vi "Newmark-CatchCharacters.vi"(0 "Table VRN IN":refnum<visa-resource-name>, 2 "Bool Refnum":refnum<vi>, 11 "Error IN":errorcluster) -> (4 "Table VRN OUT":refnum<visa-resource-name>, 6 "n_chars":u32, 10 "InterruptType":i32(ring) items=["Unknown"=-1, "Error"=0, "Slip/Stall"=1, "Overtravel"=2, "Done"=3, "None"=4], 15 "Error OUT":errorcluster)   [LabVIEW 2011]
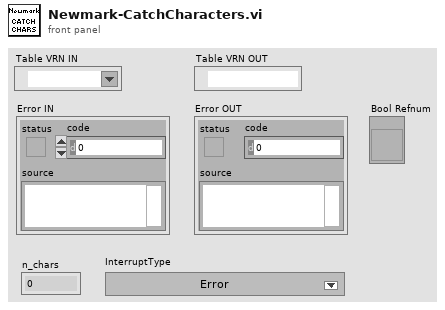
[diagram p1: front panel]
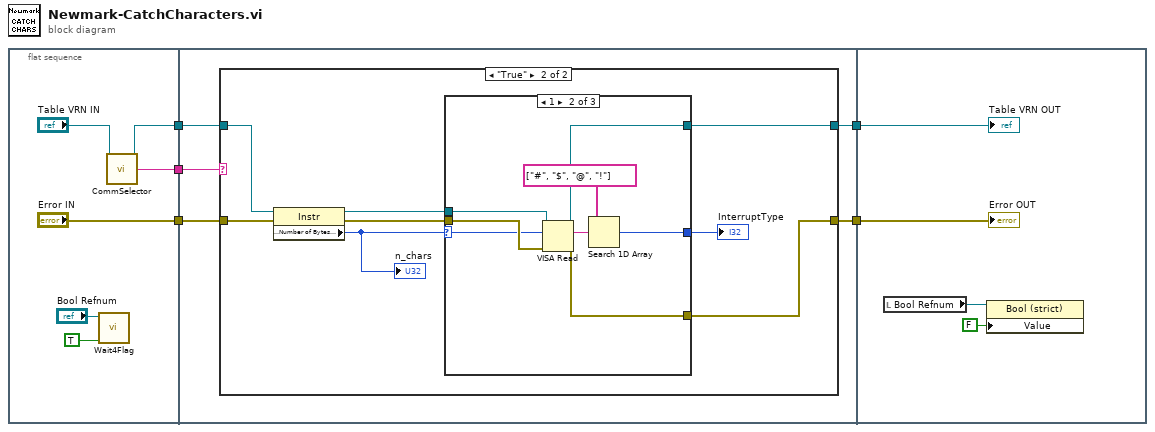
[diagram p0: block diagram]
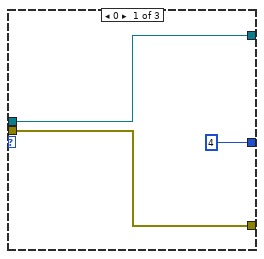
[diagram p3: hidden frame]
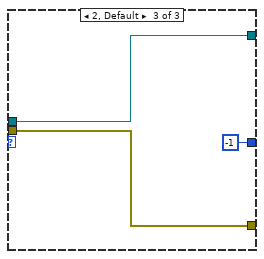
[diagram p4: hidden frame]
diagram:
  n1 = flat-sequence {
    tunnel: ["Error IN"] -> w5
    tunnel: [w7] -> w4
    tunnel: [w6] -> w3
    tunnel: w5 -> [w14]
    tunnel: w4 -> [w16]
    tunnel: w3 -> [w15]
    tunnel: [w13] -> w2
    tunnel: [w12] -> w1
    tunnel: w2 -> [w42]
    tunnel: w1 -> [w41]
    frame #0 {
      n2 = call "Wait4Flag.vi"("Raise Flag ?"=TRUE, "Ctl Refnum IN"="Bool Refnum") -> ()  [unwired: 8 in, 2 out]
      n3 = call "CommSelector.vi"("VISA resource name"="Table VRN IN") -> ("VISA resource name"=w7:refnum<visa-resource-name>, "CommType"=w6:string)  [unwired: 13 in]
    }
    frame #1 {
      n4 = case shown="\"True\"" w15 {
        tunnel: w16 -> [w18 w26]
        tunnel: w14 -> [w17 w25]
        tunnel: [w18 w20] -> w13
        tunnel: [w17 w19] -> w12
        frame "False", Default {
        }
        frame "True" {
          n5 = property on="Property Node" class="Instr"(reference=w26, error in=w25) -> (reference out=w23:refnum<visa-resource-name>, error out=w24:errorcluster, "Serial Settings:Number of Bytes at Serial Port"=w21:u32)
          "n_chars" <- w21
          n6 = case shown="1" w21 {
            selector: w21 -> [_ w33 _]
            tunnel: w24 -> [w27 w34 w38]
            tunnel: w23 -> [w28 w35 w39]
            tunnel: [4 ("index of element") w32 -1 ("index of element")] -> w22
            tunnel: [w28 w31 w39] -> w20
            tunnel: [w27 w30 w38] -> w19
            frame 0 {
            }
            frame 1 {
              n7 = VISA Read(VISA resource name=w35, byte count=w33, error in (no error)=w34) -> (VISA resource name out=w31:refnum<visa-resource-name>, read buffer=w36:string, error out=w30:errorcluster)  [unwired: 1 out]
              n8 = Search 1D Array(1D array=string[] ["#", "$", "@", "!"], element=w36) -> (index of element=w32:i32)  [unwired: 1 in]
            }
            frame 2, Default {
            }
          }
          "InterruptType" <- w22
        }
      }
    }
    frame #2 {
      n9 = local read "Bool Refnum"() -> (w44:refnum<vi>)
      n10 = property class="Bool (strict)"(reference=w44, "Value"=FALSE) -> ()  [unwired: 1 in, 2 out]
      "Table VRN OUT" <- w42
      "Error OUT" <- w41
    }
  }
